vi "ProdaNG.Example.AddProduct.vi"() -> ()   [LabVIEW 2016]
uses:
  Controls/ProdaNG.Product.ctl
  Controls/ProdaNG.Identification.ctl
panel:
  out "Identification":T1
  out "Product out 1":T2
  out "source":string
  in  "serialNumber 1":dbl=3.0
  in  "systemName":string="T10"
  out "ErrCode":i32
  out "error out":errorcluster
  in  "error in (no error)":errorcluster
  in  "wabcoNumber":string="4154064040"
  out "DataBase time":string
  in  "Connection string":string="lcptb/lcptb@PRODA_WPK"
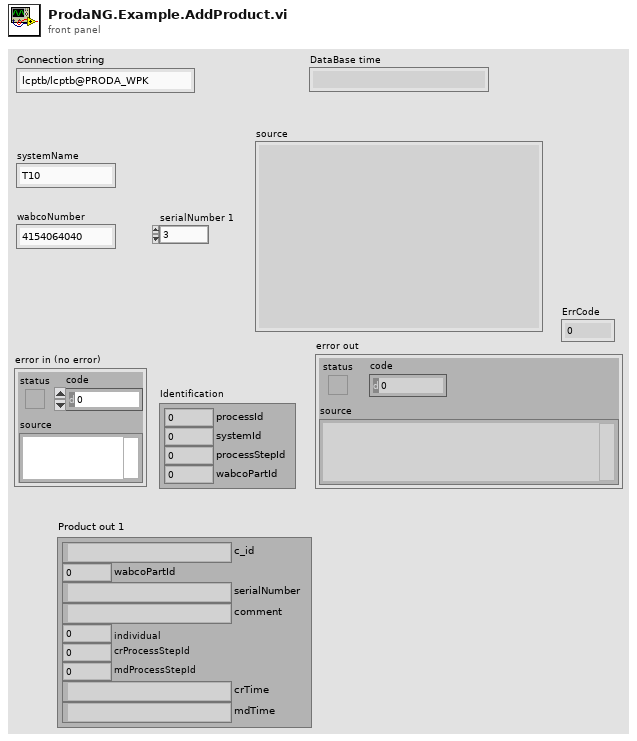
[diagram p1: front panel]
types:
  T1 = typedef "ProdaNG.Identification.ctl" = cluster{"processId":i32, "systemId":i32, "processStepId":i32, "wabcoPartId":i32}
  T2 = typedef "ProdaNG.Product.ctl" = cluster{"c_id":string, "wabcoPartId":i32, "serialNumber":string, "comment":string, "individual":i32, "crProcessStepId":i32, "mdProcessStepId":i32, "crTime":string, "mdTime":string}
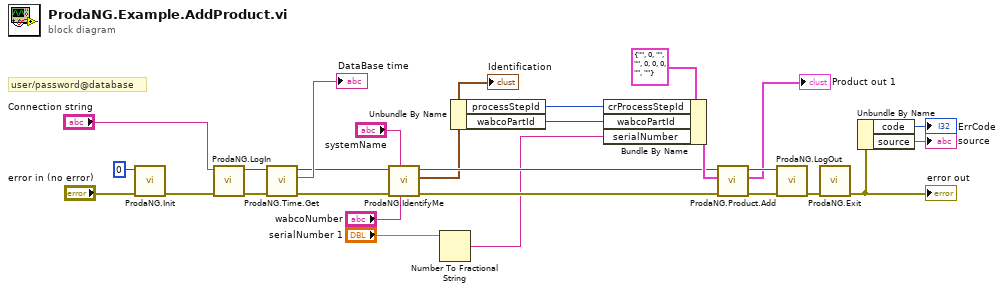
[diagram p0: block diagram]
diagram:
  # "user/password@database"
  n1 = call "ProdaNG.Init.vi"("error in (no error)"="error in (no error)", "numContexts (0: unlimited)"=0 ("numContexts")) -> ("error out"=w26:errorcluster)  [unwired: 9 in]
  n2 = call "ProdaNG.LogIn.vi"("error in"=w26, "ConnectionString"="Connection string") -> ("error out"=w22:errorcluster, "dbHandle"=w23:i32)  [unwired: 7 in, 1 out]
  n3 = call "ProdaNG.Time.Get.vi"("error in"=w22, "dbHandleIn"=w23) -> ("error out"=w17:errorcluster, "timeStr"=→"DataBase time":string, "dbHandle"=w18:i32)  [unwired: 5 in, 1 out]
  n4 = call "ProdaNG.IdentifyMe.vi"("wabcoNumber"="wabcoNumber", "systemName"="systemName", "error in"=w17, "dbHandleIn"=w18) -> ("error out"=w7:errorcluster, "Identification"=w1:T1, "dbHandle"=w10:i32)  [unwired: 5 in]
  "Identification" <- w1
  n5 = Number To Fractional String(number="serialNumber 1") -> (F-format string=w2:string)  [unwired: 2 in, 1 out]
  n6 = Unbundle By Name(w1) -> ("processStepId"=w4:i32, "wabcoPartId"=w5:i32)
  n7 = Bundle By Name(cluster=T2 {"c_id"="", "wabcoPartId"=0, "serialNumber"="", "comment"="", "individual"=0, "crProcessStepId"=0, "mdProcessStepId"=0, "crTime"="", "mdTime"=""} ("Product"), "crProcessStepId"=w4, "wabcoPartId"=w5, "serialNumber"=w2) -> (w11:T2)
  n8 = call "ProdaNG.Product.Add.vi"("error in (no error)"=w7, "Product"=w11, "dbHandle"=w10) -> ("error out"=w8:errorcluster, "Product out"=→"Product out 1":T2, "dbHandle"=w9:i32)  [unwired: 6 in]
  n9 = call "ProdaNG.LogOut.vi"("error in"=w8, "dbHandleIn"=w9) -> ("error out"=w27:errorcluster)  [unwired: 9 in]
  n10 = call "ProdaNG.Exit.vi"("error in (no error)"=w27) -> ("error out"=w13:errorcluster)  [unwired: 10 in]
  "error out" <- w13
  n11 = Unbundle By Name(w13) -> ("code"=→"ErrCode":i32, "source"=→"source":string)
